vi "VI Control - Get All Control References.vi"(7 "Control References - Top Level":refnum<vi>[](array[refnum])) -> (8 "Control References - Complete":refnum<vi>[](array[refnum]), 10 "Control Names":string[](array[string]), 15 "error out":errorcluster)   [LabVIEW 2011]
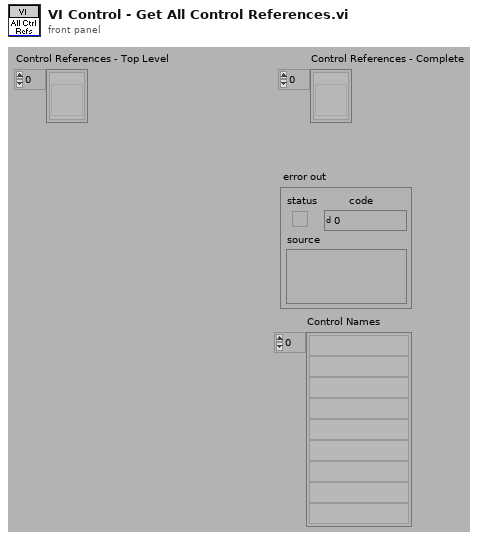
[diagram p1: front panel]
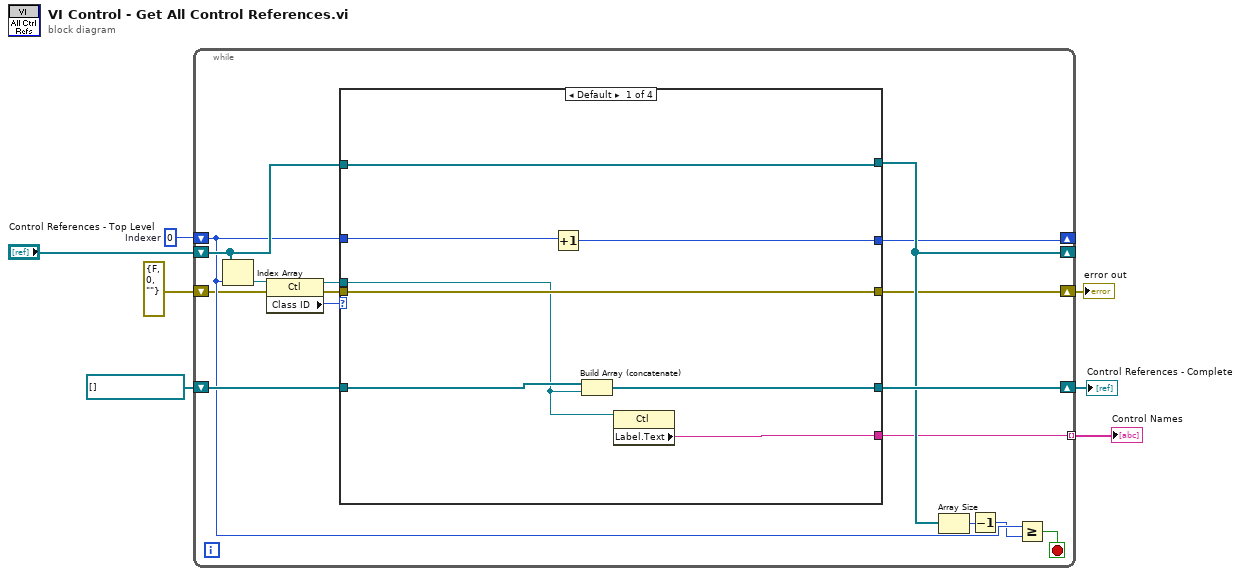
[diagram p0: block diagram]
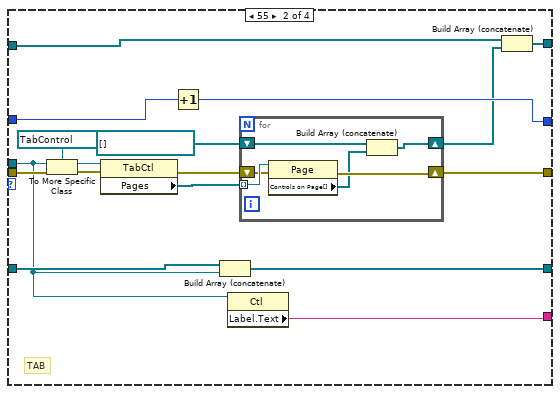
[diagram p2: hidden frame]
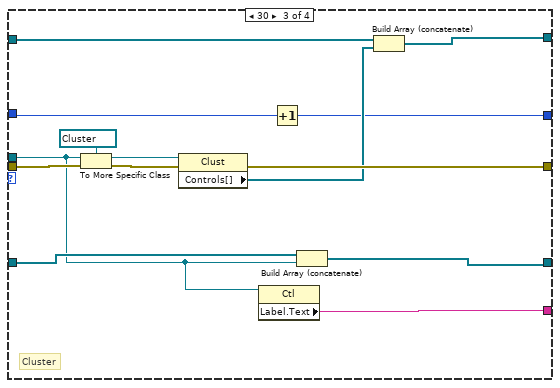
[diagram p3: hidden frame]
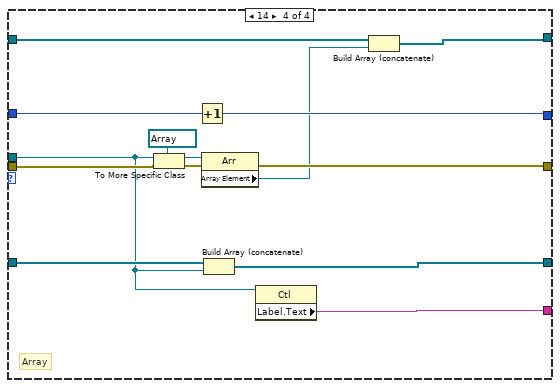
[diagram p4: hidden frame]
diagram:
  w5 = 0  # Indexer
  n1 = while {
    shift-right: [w21] -> w2
    shift-left: refnum<vi>[] [] -> [w22]
    shift-right: [w16] -> _
    shift-left: "Control References - Top Level" -> [w19]
    shift-right: [w15] -> _
    shift-left: w5 -> [w14]
    shift-right: [w12] -> w4
    shift-left: errorcluster {"status"=FALSE, "code"=0, "source"=""} ("error in") -> [w13]
    tunnel: [w8] -> w1 mode=indexing
    stop <- w17 stop-if-true
    n2 = Index Array(array=w19, index=w14) -> (element=w20:refnum<vi>)
    n3 = property class="Ctl"(reference=w20, error in=w13) -> (reference out=w23:refnum<vi>, error out=w11:errorcluster, "Class ID"=w9:u32)
    n4 = case shown="Default" w9 {
      tunnel: w23 -> [w25 w33 w56 w70]
      tunnel: w22 -> [w26 w34 w60 w72]
      tunnel: [w31 w41 w61 w71] -> w21
      tunnel: [w30 w45 w68 w79] -> w16
      tunnel: w19 -> [w30 w43 w58 w80]
      tunnel: w14 -> [w29 w40 w59 w78]
      tunnel: [w28 w44 w57 w81] -> w15
      tunnel: w11 -> [w27 w38 w66 w76]
      tunnel: [w27 w35 w64 w74] -> w12
      tunnel: [w24 w32 w55 w69] -> w8
      frame Default {
        n5 = Increment(x=w29) -> (x+1=w28:i32)
        n6 = Build Array (concatenate)(w26, w25) -> (w31:refnum<vi>[])
        n7 = property class="Ctl"(reference=w25) -> ("Label.Text"=w24:string)  [unwired: 1 in, 2 out]
      }
      frame 55 {
        # "TAB"
        n8 = To More Specific Class(target class=refnum<vi> refnum ("TabCtl Refnum"), reference=w33, error in=w38) -> (specific class reference=w47:refnum<vi>, error out=w37:errorcluster)
        n9 = property class="TabCtl"(reference=w47, error in=w37) -> (error out=w36:errorcluster, "Pages"=w48:refnum<vi>[])  [unwired: 1 out]
        n10 = Increment(x=w40) -> (x+1=w44:i32)
        n11 = Build Array (concatenate)(w34, w33) -> (w41:refnum<vi>[])
        n12 = property class="Ctl"(reference=w33) -> ("Label.Text"=w32:string)  [unwired: 1 in, 2 out]
        n13 = for {
          tunnel: w48 -> [w54] mode=indexing
          shift-right: [w52] -> w42
          shift-left: refnum<vi>[] [] -> [w53]
          shift-right: [w50] -> w35
          shift-left: w36 -> [w51]
          n14 = property class="Page"(reference=w54, error in=w51) -> (error out=w50:errorcluster, "Controls on Page[]"=w49:refnum<vi>[])  [unwired: 1 out]
          n15 = Build Array (concatenate)(w53, w49) -> (w52:refnum<vi>[])
        }
        n16 = Build Array (concatenate)(w43, w42) -> (w45:refnum<vi>[])
      }
      frame 30 {
        # "Cluster"
        n17 = To More Specific Class(target class=refnum<vi> refnum ("Clust Refnum"), reference=w56, error in=w66) -> (specific class reference=w62:refnum<vi>, error out=w65:errorcluster)
        n18 = property class="Clust"(reference=w62, error in=w65) -> (error out=w64:errorcluster, "Controls[]"=w63:refnum<vi>[])  [unwired: 1 out]
        n19 = property class="Ctl"(reference=w56) -> ("Label.Text"=w55:string)  [unwired: 1 in, 2 out]
        n20 = Increment(x=w59) -> (x+1=w57:i32)
        n21 = Build Array (concatenate)(w60, w56) -> (w61:refnum<vi>[])
        n22 = Build Array (concatenate)(w58, w63) -> (w68:refnum<vi>[])
      }
      frame 14 {
        # "Array"
        n23 = To More Specific Class(target class=refnum<vi> refnum ("Array Refnum"), reference=w70, error in=w76) -> (specific class reference=w82:refnum<vi>, error out=w75:errorcluster)
        n24 = Increment(x=w78) -> (x+1=w81:i32)
        n25 = property class="Arr"(reference=w82, error in=w75) -> (error out=w74:errorcluster, "Array Element"=w73:refnum<vi>)  [unwired: 1 out]
        n26 = Build Array (concatenate)(w72, w70) -> (w71:refnum<vi>[])
        n27 = property class="Ctl"(reference=w70) -> ("Label.Text"=w69:string)  [unwired: 1 in, 2 out]
        n28 = Build Array (concatenate)(w80, w73) -> (w79:refnum<vi>[])
      }
    }
    n29 = Array Size(array=w16) -> (size(s)=w18:i32)
    n30 = Decrement(x=w18) -> (x-1=w10:i32)
    n31 = Greater Or Equal?(x=w14, y=w10) -> (x >= y?=w17:bool)
  }
  "Control References - Complete" <- w2
  "error out" <- w4
  "Control Names" <- w1
